vi "SVL Running RMS Level (resampled) (N Ch).vi"(6 "restart averaging (F)":bool, 8 "error in (no error)":errorcluster, 9 "integration revolutions":dbl=1.0 format="%.2f", 10 "even-angle channel info":T1[](array[typedef]) {"channel info"."pregain" format="%.2f"; "channel info"."weighting filter" items=["Linear", "A-weighting", "B-weighting", "C-weighting", "ITU-R 468-4", "Dolby", "CCITT", "C-message", "Wb", "Wc", "Wd", "We", "Wf", "Wh", "Wj", "Wk", "Wm", "AES17 20 kHz lowpass", "AES17 40 kHz lowpass", "AES17 20 kHz highpass", "AES17 40 kHz highpass"]; "channel info"."dB reference" format="%^.1e"; "channel info"."engineering units" items=["custom..."=0, "V"=1, "A"=21, "C"=30, "pC"=31, "s"=32, "-"=29, "Pa"=2, "N"=20, "g"=3, "m/s^2"=4, "m/s"=5, "m"=6, "mm/s"=12, "mm"=13, "micron/s"=14, "micron"=15, "in/s^2"=7, "in/s"=8, "in"=9, "mil/s"=10, "mil"=11, "rad/s^2"=16, "rad/s"=17, "rad"=18, "deg/s^2"=26, "deg/s"=27, "deg"=28, "RPM"=22, "cycle/s^2"=23, "Hz"=24, "cycle"=25, "strain"=19]; "channel info"."sensor sensitivity" format="%#_5f"}, 11 "even-angle signals [EU]":T5(array[cluster]) {"even-angle signal" format="%.2f"; "dr" format="%.2f"; "r0" format="%.2f"}) -> (0 "error out":errorcluster, 1 "actual integration revolutions":dbl=nan format="%.2f", 2 "unit labels":string[](array[string]), 3 "running RMS levels [EU rms]":dbl[](array[numeric])=[nan] format="%.2f")   [LabVIEW 2017, in "SoundVib_VibrationLevel.lvlib"]
doc: "Computes the running root-mean-square (RMS) level of <B>scaled signal [EU]</B> or <B>even-angle signal [EU]</B>. <B>scaled signal [EU]</B> should have a zero DC component. You can attenuate the DC component with hardware AC-coupling filters and with software high-pass filters. <B>integration time [s]</B> and <B>integration revolutions</B> specify the duration over which the RMS level is computed. A new running RMS value is returned each time you call this VI. A shift register internal to this VI maintains the result of past runs. The new result is an averaged level that includes the latest block of samples and the level history in the specified integration time. Wire data to the <B>scaled signal [EU]</B> input to determine the polymorphic instance to use or manually select the instance."
uses:
  <vilib>/addons/Sound and Vibration/svt_Level/SoundVib_VibrationLevel.lvlib
  <vilib>/addons/_NISVFA/_Shared subVIs/Controls/svc_Resampled Channel Info.ctl
  <vilib>/addons/_NISVFA/_Shared subVIs/Controls/svc_Channel Info.ctl
  <vilib>/addons/_NISVFA/_Shared subVIs/Controls/svc_Engineering Units Text Ring.ctl
  <vilib>/addons/_NISVFA/_Shared subVIs/Controls/svc_Weighting Filter Text Ring.ctl
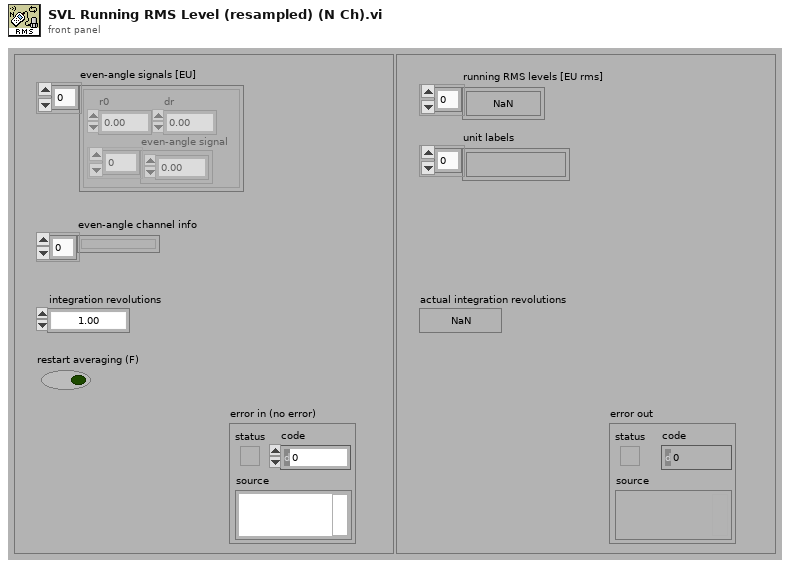
[diagram p1: front panel]
types:
  T1 = typedef "svc_Resampled Channel Info.ctl" = cluster{"channel name":string, "description":string, " channel info":T2}
  T2 = typedef "svc_Channel Info.ctl" = cluster{"sensor sensitivity":dbl, "engineering units":T3, "dB reference":dbl, "custom label":string, "weighting filter":T4, "pregain":dbl}
  T3 = typedef "svc_Engineering Units Text Ring.ctl" = u16
  T4 = typedef "svc_Weighting Filter Text Ring.ctl" = u16
  T5 = cluster{"r0":dbl, "dr":dbl, "even-angle signal":dbl[]}[]
  T6 = enum16{"RMS", "Running RMS", "Exp avg  ", "Dec exp avg ", "Peak", "Crest"}
  T7 = cluster{"r0":dbl, "dr":dbl, "even angle signal":dbl[]}[]
  T8 = enum16{"Reset filter", "Restart averaging", "Continue processing"}
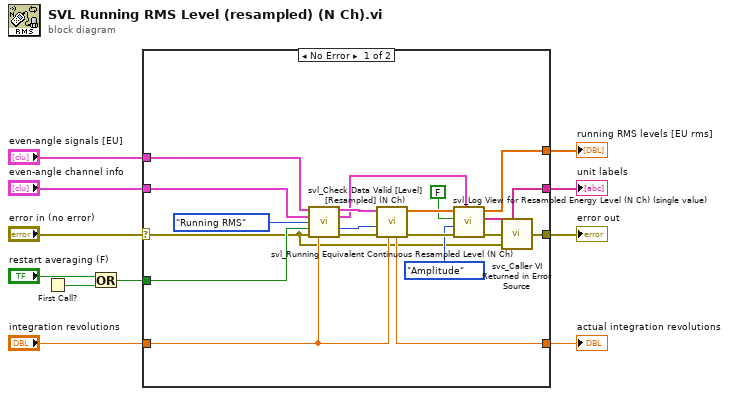
[diagram p0: block diagram]
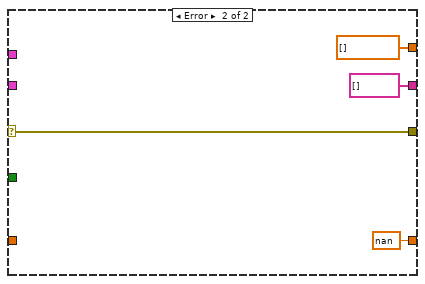
[diagram p2: hidden frame]
diagram:
  n1 = First Call?() -> (First Call?: T/F=w5:bool)
  n2 = Or(x="restart averaging (F)", y=w5) -> (x .or. y?=w3:bool)
  n3 = case shown="No Error" "error in (no error)" {
    selector: "error in (no error)" -> [w12 w34]
    tunnel: [w23 w34] -> w11
    tunnel: [w22 nan ("actual integration time [s]")] -> w10
    tunnel: [w27 dbl[] [] ("energy levels [EU^2 rms]")] -> w9
    tunnel: [w26 string[] [] ("unit label [ ]")] -> w8
    tunnel: "integration revolutions" -> [w18 _]
    tunnel: "even-angle signals [EU]" -> [w14 _]
    tunnel: w3 -> [w20 _]
    tunnel: "even-angle channel info" -> [w13 _]
    frame No Error {
      n4 = call <vilib>:"svl_Check Data Valid [Level] [Resampled] (N Ch).vi"("scaled even angle signals [EU]"=w14, "even angle channel info"=w13, "level analysis"=T6."Running RMS" ("Level Analysis"), "restart averaging (F)"=w20, "error in (no error)"=w12, "integration time [s]"=w18) -> ("dup scaled even angle signals [EU]"=w16:T7, "dup even angle channel info"=w15:T1[], "processing state"=w19:T8, "error out"=w21:errorcluster)  [unwired: 6 in]
      n5 = call <vilib>:"svl_Running Equivalent Continuous Resampled Level (N Ch).vi"("integration time [s]"=w18, "error in (no error)"=w21, "processing state"=w19, "scaled signals [EU]"=w16) -> ("error out"=w29:errorcluster, "energy level [ ] [EU^2 rms]"=w30:dbl[], "actual integration time [s]"=w22:dbl)  [unwired: 5 in]
      n6 = call <vilib>:"svl_Log View for Resampled Energy Level (N Ch) (single value).vi"("even angle channel info"=w15, "error in (no error)"=w29, "view mode"=enum16{"Power", "Amplitude"}."Amplitude", "dB On (T)"=FALSE, "energy levels [EU^2 rms]"=w30) -> ("error out"=w28:errorcluster, "unit label [ ]"=w26:string[], "energy levels [EU^2 rms]"=w27:dbl[])  [unwired: 4 in]
      n7 = call <vilib>:"svc_Caller VI Returned in Error Source.vi"("warning input to caller"=w12, "error in (no error)"=w28) -> ("error out"=w23:errorcluster)  [unwired: 3 in]
    }
    frame Error {
    }
  }
  "running RMS levels [EU rms]" <- w9
  "unit labels" <- w8
  "actual integration revolutions" <- w10
  "error out" <- w11
